vi "LibXML_CheckNodeEmpty.vi"(8 "error in":errorcluster, 10 "node in":u32) -> (0 "error out":errorcluster, 2 "blankNode!":bool)   [LabVIEW 2019, in "Tools.lvlib" / "LibXML.lvlib"]
uses:
  LibXML.lvlib
  dll/libxml2.dll
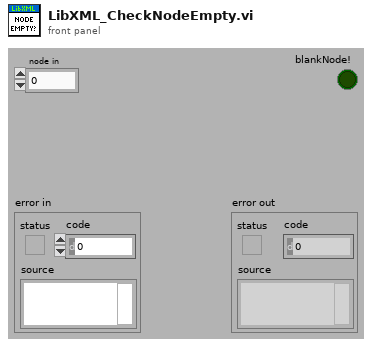
[diagram p1: front panel]
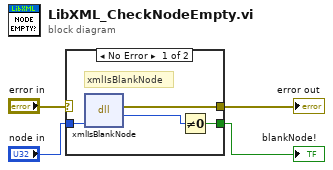
[diagram p0: block diagram]
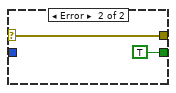
[diagram p2: hidden frame]
diagram:
  n1 = case shown="No Error" "error in" {
    selector: "error in" -> [_ w10]
    tunnel: [w7 w10] -> w3
    tunnel: [w6 TRUE] -> w2
    tunnel: "node in" -> [w5 _]
    frame No Error {
      # "xmlIsBlankNode"
      n2 = dll-call lib="C:/Projects/_Prywatne/MyCIT/Framework/Tools/XML/LibXML/dll/libxml2.dll" fn="xmlIsBlankNode"("node"=w5) -> (error out=w7:errorcluster, "return type"=w8:u32)  [unwired: 4 in, 1 out]
      n3 = Not Equal To 0?(x=w8) -> (x != 0?=w6:bool)
    }
    frame Error {
    }
  }
  "error out" <- w3
  "blankNode!" <- w2
